vi "Single Float Value.vi"(8 "error in (no error)":errorcluster, 11 "Double Float in":refnum<class "Abs_I64 Integer.lvclass">) -> (0 "error out":errorcluster, 2 "Float":sgl, 3 "Double Float out":refnum<class "Abs_I64 Integer.lvclass">)   [LabVIEW 2021, in "Abs_I64 Integer.lvclass"]
uses:
  Abs_I64 Integer.lvclass
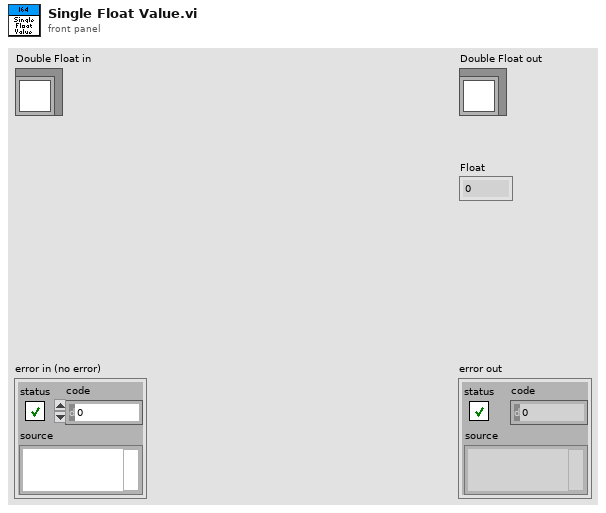
[diagram p1: front panel]
types:
  T1 = typedef "Abs_I64 Integer.lvclass/Type.ctl" = i64
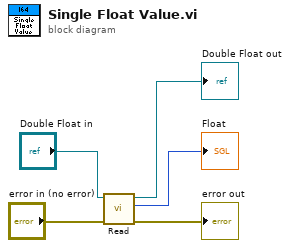
[diagram p0: block diagram]
diagram:
  n1 = call-dynamic "Read.vi"("error in (no error)"="error in (no error)", "Double Float.lvclass_340760 in"="Double Float in") -> ("error out"=→"error out":errorcluster, "Value"=→"Float":T1, "Double Float.lvclass_340760 out"=→"Double Float out":refnum<class "Abs_I64 Integer.lvclass">)  [unwired: 7 in]
